vi "MSScript transcoder.vi"(8 "error in (no error)":errorcluster, 11 "new value":variant) -> (0 "error out":errorcluster, 3 "script code":string)   [LabVIEW 2018]
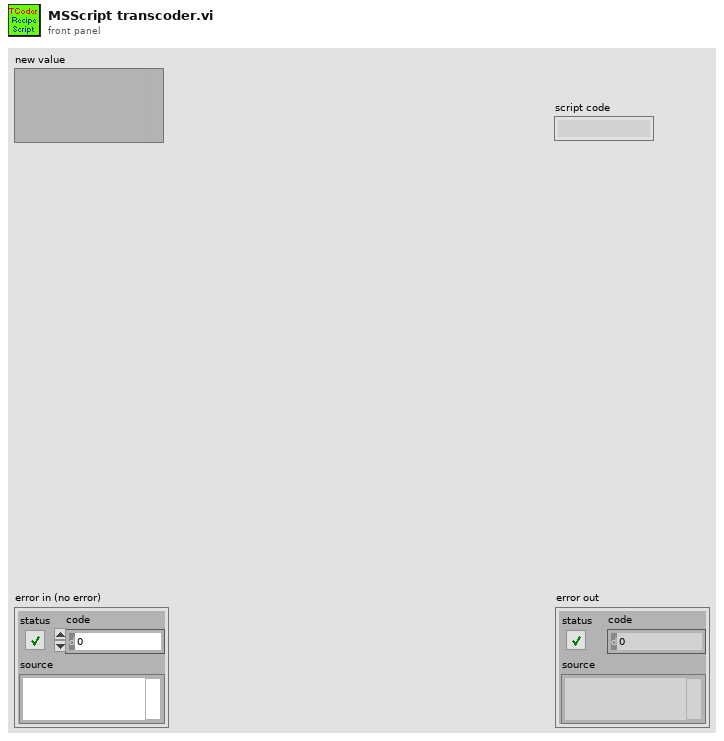
[diagram p1: front panel]
types:
  T1 = cluster{"param":cluster{"label":string, "data":string}[], "code":string}
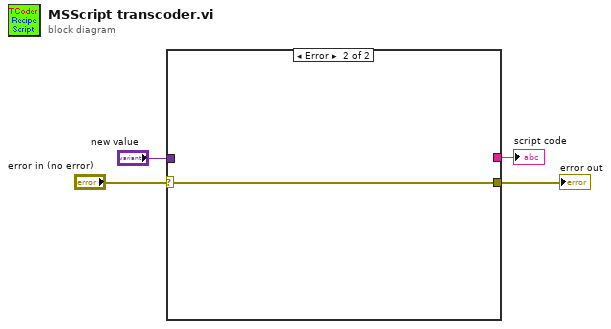
[diagram p0: block diagram]
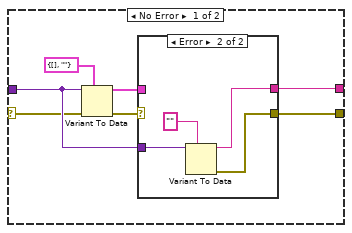
[diagram p2: hidden frame]
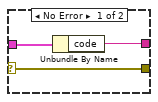
[diagram p3: hidden frame]
diagram:
  n1 = case shown="Error" "error in (no error)" {
    selector: "error in (no error)" -> [w7 w19]
    tunnel: "new value" -> [w8 _]
    tunnel: [w6 w19] -> w2
    tunnel: [w5 _] -> w1
    frame No Error {
      n2 = Variant To Data(error in=w7, type=T1 {"param"=[], "code"=""} ("Script"), Variant=w8) -> (data=w9:T1, error out=w10:errorcluster)
      n3 = case shown="Error" w10 {
        selector: w10 -> [w14 _]
        tunnel: [w14 w17] -> w6
        tunnel: w8 -> [_ w16]
        tunnel: w9 -> [w13 _]
        tunnel: [w12 w15] -> w5
        frame No Error {
          n4 = Unbundle By Name(w13) -> ("code"=w12:string)
        }
        frame Error {
          n5 = Variant To Data(type="", Variant=w16) -> (data=w15:string, error out=w17:errorcluster)  [unwired: 1 in]
        }
      }
    }
    frame Error {
    }
  }
  "error out" <- w2
  "script code" <- w1
